vi "Initialise.vi"(8 "error in (no error)":errorcluster, 10 "Message in":refnum<class "InitialiseMessage.lvclass">, 11 "DAQMH121119OrcaFlash in":refnum<class "DAQOrcaFlash.lvclass">) -> (0 "error out":errorcluster, 3 "DAQMH121119OrcaFlash out":refnum<class "DAQOrcaFlash.lvclass">)   [LabVIEW 2012, in "DAQOrcaFlash.lvclass"]
doc: "This member function is called when the statemachine in the run.vi receives an 'initialise' message. It mainly initialises the RabbitMQ connectivity. \n\nOverride this member function in your derived class to initialise hardware or software resources (but don't forget to call the parent method). If your component owns subcomponents, they count as resources, so you have to initialise them by calling their own initialise functions."
uses:
  DAQOrcaFlash.lvclass
  <vilib>/Distrio/Murmex/InitialiseMessage/InitialiseMessage.lvclass
  <vilib>/Distrio/Murmex/Murmex/Murmex.lvclass
  <vilib>/Distrio/Murmex/TerminateMessage/TerminateMessage.lvclass
  <vilib>/Distrio/Murmex/UpdateMessage/UpdateMessage.lvclass
  DAQOrcaFlash.lvclass/DAQOrcaFlash.ctl
panel:
  # "This method is called when the INTIALISE\ntrigger is sent. \n\nOverride this method when your component needs to\nrespond to this trigger. \n\nCall parent for proper implementation"
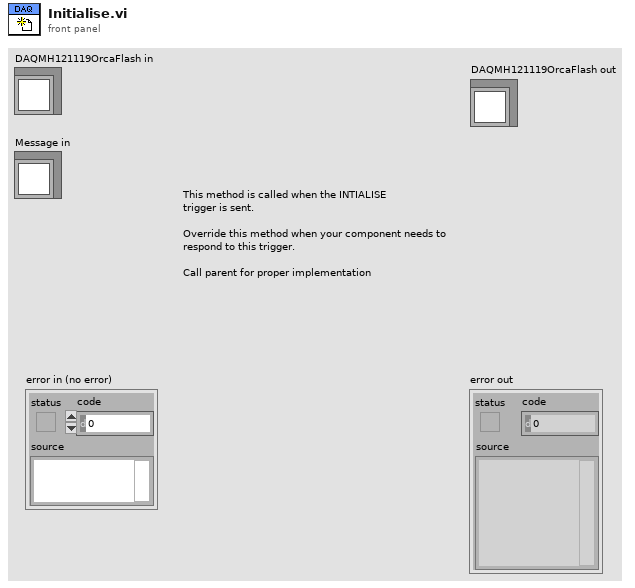
[diagram p1: front panel]
types:
  T1 = cluster{"Mode":u32, "Polarity":u32, "Period":dbl, "Delay":dbl}
  T2 = typedef "Image Type" = u32
  T3 = typedef "IMAQ Image.ctl" = refnum<image>
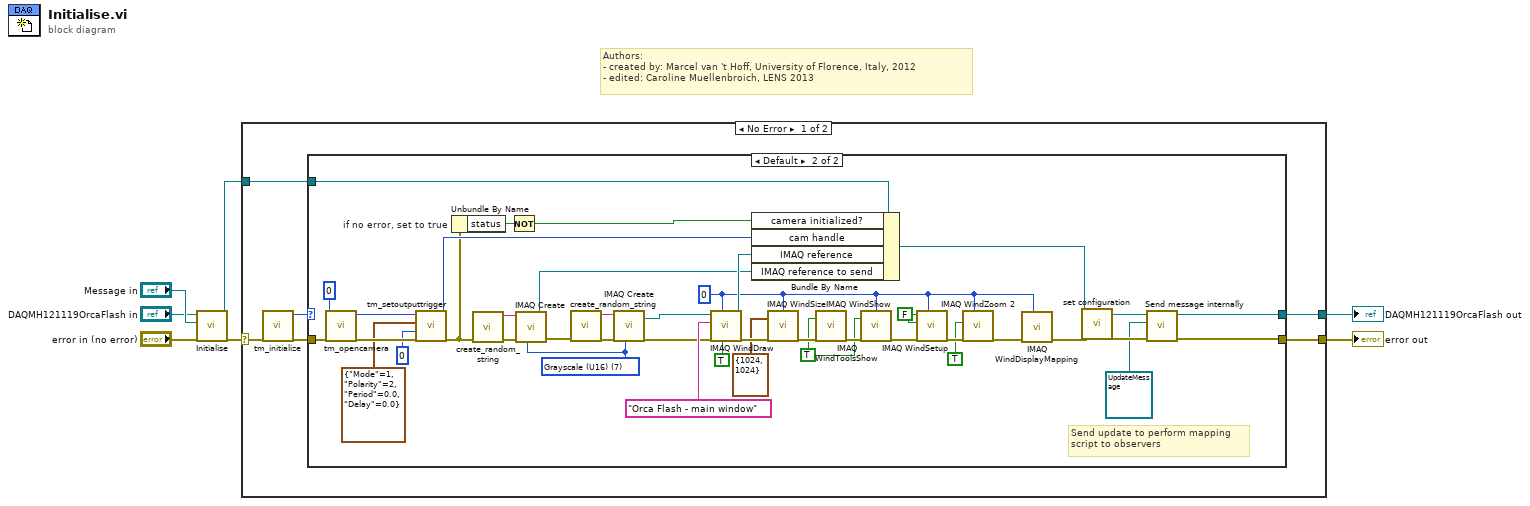
[diagram p0: block diagram]
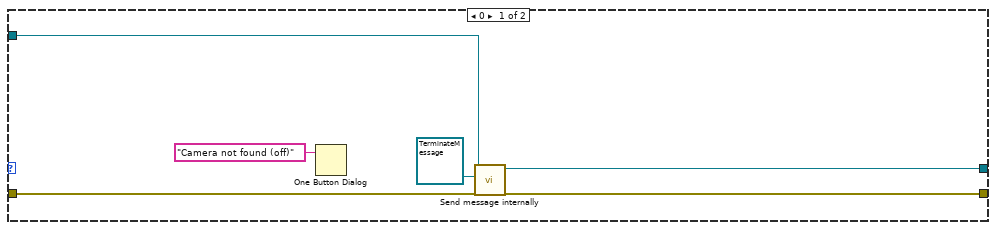
[diagram p2: hidden frame]
diagram:
  # "Authors: \n- created by: Marcel van 't Hoff, University of Florence, Italy, 2012\n- edited: Caroline Muellenbroich, LENS 2013"
  n1 = call-parent "Initialise.vi"("error in (no error)"="error in (no error)", "Message in"="Message in", "Murmex in"="DAQMH121119OrcaFlash in") -> ("error out"=w4:errorcluster, "Murmex out"=w3:refnum<class "DAQOrcaFlash.lvclass">)  [unwired: 7 in]
  n2 = case shown="No Error" w4 {
    selector: w4 -> [w12 w61]
    tunnel: w3 -> [w11 w62]
    tunnel: [w10 w62] -> w2
    tunnel: [w9 w61] -> w1
    frame No Error {
      n3 = call <userlib>:"tm_initialize.vi"("error in (no error)"=w12) -> ("error out"=w13:errorcluster, "Number Of Cameras"=w8:u32)  [unwired: 9 in]
      n4 = case shown="Default" w8 {
        tunnel: w13 -> [w19 w60]
        tunnel: w11 -> [w17 w56]
        tunnel: [w16 w27] -> w10
        tunnel: [w18 w29] -> w9
        frame 0 {
          n5 = One Button Dialog(message="Camera not found (off)") -> ()  [unwired: 1 in, 1 out]
          n6 = call <vilib>:"Send message internally.vi"("error in (no error)"=w19, "Message"=refnum<class "TerminateMessage.lvclass"> refnum ("TerminateMessage"), "Murmex in"=w17) -> ("error out"=w18:errorcluster, "Murmex out"=w16:refnum<class "DAQOrcaFlash.lvclass">)  [unwired: 7 in]
        }
        frame Default {
          w44 = FALSE ("Window can grow? (Yes)")
          w20 = 0 ("Window Number (0...15)")
          w46 = TRUE ("Hide/Show (Show)")
          w33 = T2 7 items=["Grayscale (U8)", "Grayscale (I16)", "Grayscale (SGL)", "Complex (CSG)", "RGB (U32)", "HSL (U32)", "RGB (U64)", "Grayscale (U16)"] ("Image Type")
          # "Send update to perform mapping\nscript to observers"
          n7 = call <userlib>:"tm_opencamera.vi"("error in (no error)"=w60, "Camera Index"=u32 0) -> ("error out"=w40:errorcluster, "Handle out"=w41:u32)  [unwired: 8 in]
          n8 = call <userlib>:"tm_setoutputtrigger.vi"("error in (no error)"=w40, "Index"=0, "Parameters"=T1 {"Mode"=1, "Polarity"=2, "Period"=0.0, "Delay"=0.0}, "Handle in"=w41) -> ("error out"=w25:errorcluster, "Handle out"=w37:u32)  [unwired: 6 in]
          n9 = Unbundle By Name "if no error, set to true"(w25) -> ("status"=w24:bool)
          n10 = call "create_random_string.vi"("error in (no error)"=w25) -> ("error out"=w34:errorcluster, "random string"=w32:string)  [unwired: 9 in]
          n11 = Not(x=w24) -> (.not. x?=w23:bool)
          n12 = call "IMAQ Create"("Image Name"=w32, "Image Type"=w33, "error in (no error)"=w34) -> ("New Image"=w31:T3, "error out"=w35:errorcluster)  [unwired: 2 in]
          n13 = call "create_random_string.vi"("error in (no error)"=w35) -> ("error out"=w58:errorcluster, "random string"=w57:string)  [unwired: 9 in]
          n14 = call "IMAQ Create"("Image Name"=w57, "Image Type"=w33, "error in (no error)"=w58) -> ("New Image"=w53:T3, "error out"=w50:errorcluster)  [unwired: 2 in]
          n15 = call "IMAQ WindDraw"("Resize to Image Size? (Y)"=TRUE, "Window Number (0...15)"=w20, "error in (no error)"=w50, "Title"="Orca Flash - main window", "Image"=w53) -> ("error out"=w49:errorcluster, "Image Out (duplicate)"=w54:T3)  [unwired: 5 in]
          n16 = Bundle By Name(cluster=w56, "camera initialized?"=w23, "cam handle"=w37, "IMAQ reference"=w54, "IMAQ reference to send"=w31) -> (w36:refnum<class "DAQOrcaFlash.lvclass">)
          n17 = call "IMAQ WindSize"("error in (no error)"=w49, "Width & Height"=cluster{"Width":i32, "Height":i32} {"Width"=1024, "Height"=1024}, "Window Number"=w20) -> ("error out"=w48:errorcluster)  [unwired: 3 in, 2 out]
          n18 = call "IMAQ WindToolsShow"("Hide/Show (Show)"=w46, "error in (no error)"=w48) -> ("error out"=w55:errorcluster)  [unwired: 3 in, 1 out]
          n19 = call "IMAQ WindShow"("error in (no error)"=w55, "Hide/Show (Show)"=w46, "Window Number (0...15)"=w20) -> ("error out"=w45:errorcluster)  [unwired: 3 in, 2 out]
          n20 = call "IMAQ WindSetup"("Window Number (0...15)"=w20, "error in (no error)"=w45, "Window can close? (Yes)"=w44, "Window can grow? (Yes)"=w44) -> ("error out"=w43:errorcluster)  [unwired: 7 in]
          n21 = call "IMAQ WindZoom 2"("Window Number (0...15)"=w20, "error in (no error)"=w43, "Zoom to Fit? (False)"=TRUE) -> ("error out"=w22:errorcluster)  [unwired: 5 in, 3 out]
          n22 = call "IMAQ WindDisplayMapping"("Window Number (0...15)"=w20, "error in (no error)"=w22) -> ("error out"=w21:errorcluster)  [unwired: 8 in, 1 out]
          n23 = call-dynamic "set configuration.vi"("error in (no error)"=w21, "DAQOrcaFlash in"=w36) -> ("error out"=w30:errorcluster, "DAQOrcaFlash out"=w28:refnum<class "DAQOrcaFlash.lvclass">)  [unwired: 8 in]
          n24 = call <vilib>:"Send message internally.vi"("error in (no error)"=w30, "Message"=refnum<class "UpdateMessage.lvclass"> refnum ("Distrio Murmex 1.0:UpdateMessage"), "Murmex in"=w28) -> ("error out"=w29:errorcluster, "Murmex out"=w27:refnum<class "DAQOrcaFlash.lvclass">)  [unwired: 7 in]
        }
      }
    }
    frame Error {
    }
  }
  "error out" <- w1
  "DAQMH121119OrcaFlash out" <- w2
